vi "ARRAY TDX TO SCRIPT RTS .vi"(8 "error in (no error)":errorcluster, 11 "TDX":bool[](array[boolean])) -> (0 "error out":errorcluster, 1 "TRANSD":u64, 3 "SCRIPT OUT":string[](array[string]))   [LabVIEW 2014, in "CAP-USB.lvlib"]
doc: "Arma la trama completa de configuracion por transductor\nque debe ser enviada al CAP-USB"
uses:
  CAP-USB.lvlib
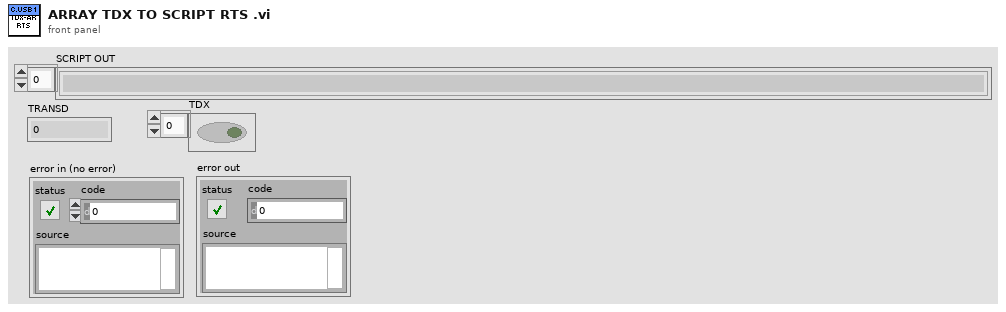
[diagram p1: front panel]
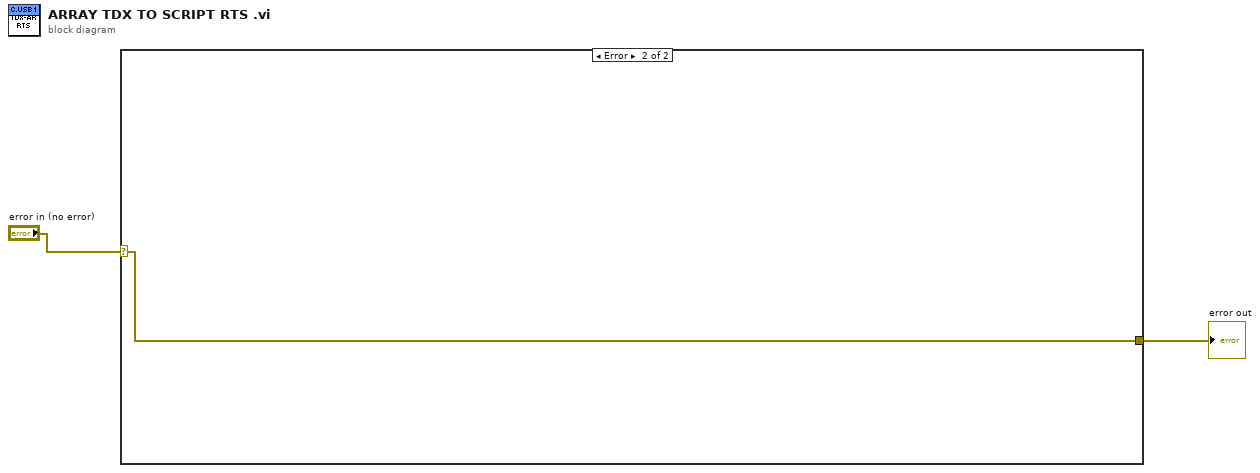
[diagram p0: block diagram]
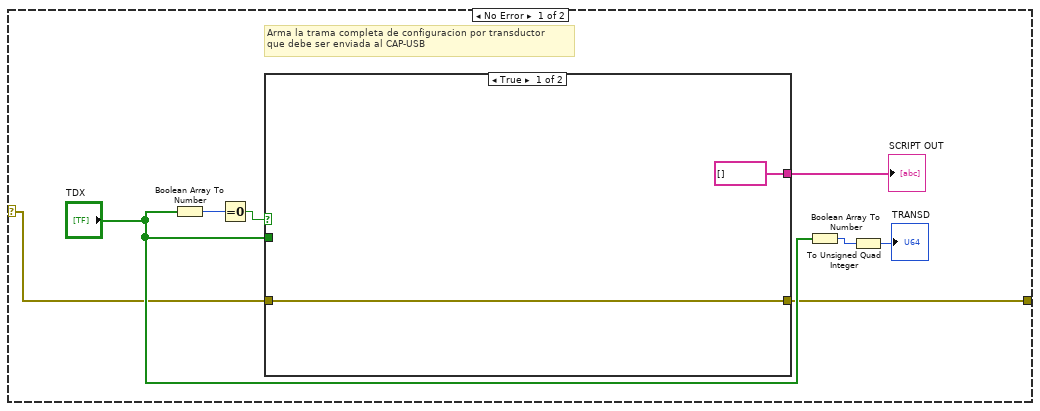
[diagram p2: hidden frame]
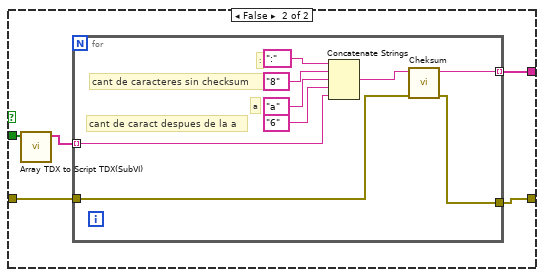
[diagram p3: hidden frame]
diagram:
  n1 = case shown="Error" "error in (no error)" {
    selector: "error in (no error)" -> [w4 w27]
    tunnel: [w3 w27] -> w1
    frame No Error {
      # "Arma la trama completa de configuracion por transductor\nque debe ser enviada al CAP-USB"
      n2 = Boolean Array To Number(Boolean array="TDX") -> (number=w9:u32)
      n3 = Equal To 0?(x=w9) -> (x = 0?=w8:bool)
      n4 = case shown="True" w8 {
        tunnel: [string[] [] w17] -> w10
        tunnel: "TDX" -> [_ w15]
        tunnel: w4 -> [w11 w14]
        tunnel: [w11 w13] -> w3
        frame True {
        }
        frame False {
          n5 = call "Array TDX to Script TDX(SubVI).vi"("TDX IN"=w15) -> ("TDX CONFIG"=w16:string[])  [unwired: 10 in]
          n6 = for {
            tunnel: w16 -> [w22] mode=indexing
            tunnel: [w20] -> w17 mode=indexing
            tunnel: w14 -> [w19]
            tunnel: [w18] -> w13
            # "cant de caract despues de la a"
            # "a"
            # "cant de caracteres sin checksum"
            # ":"
            n7 = Concatenate Strings(":" ("string"), "8" ("string"), "a" ("string"), "6" ("string"), w22) -> (w21:string)
            n8 = call "Cheksum.vi"("error in (no error)"=w19, "Trama IN"=w21) -> ("error out"=w18:errorcluster, "Trama RTS"=w20:string)  [unwired: 8 in]
          }
        }
      }
      "SCRIPT OUT" <- w10
      n9 = Boolean Array To Number(Boolean array="TDX") -> (number=w6:u32)
      n10 = To Unsigned Quad Integer(1:w6) -> (0:→"TRANSD":u64)
    }
    frame Error {
    }
  }
  "error out" <- w1
